vi "PCO_SetDelayExposureTime.vi"(6 "wTimeBaseExposure":u16(ring) items=["ns", "us", "ms"], 7 "wTimeBaseDelay":u16(ring) items=["ns", "us", "ms"], 8 "error in (no error)":errorcluster {"code" format="%x"}, 9 "dwExposure":u32, 10 "dwDelay":u32, 11 "ph":u64) -> (0 "error out":errorcluster {"code" format="%x"}, 2 "ErrorMessage":i32 format="%x", 3 "ph out":u64)   [LabVIEW 2019, in "SDK.lvlib" / "TimingControl.lvlib"]
doc: "<b>Description:</b>\nThis function does set the delay and exposure time and the associated time base values.\nWhen the Recording State of the camera is [run], camera timing is changed immediately (best possible), else new settings will be valid after a call of PCO_ArmCamera.\nRestrictions for the parameter values are defined through the following values in the camera description PCO_Description structure: dwMinDelayDESC, dwMaxDelayDESC, dwMinDelayStepDESC, dwMinExposDESC, dwMaxExposDESC, dwMinExposStepDESC\nDue to hardware limitations the input values cannot be set exactly for the pco.edge, pco.dimax and pco.1300 and therefore are changed to the next possible values in the camera. To retrieve the exact timing values, which are used in the pco.edge, please use function PCO_GetImageTiming.\nBecause frame rate and exposure time are also affected by the PCO_SetFrameRate command, it is strongly recommended to use either the PCO_SetFrameRate or the PCO_SetDelayExposureTime command.\n\n<b>Supported camera type:</b>\nAll cameras\n\n<b>Descriptor dependency:</b>\nNone"
uses:
  TimingControl.lvlib
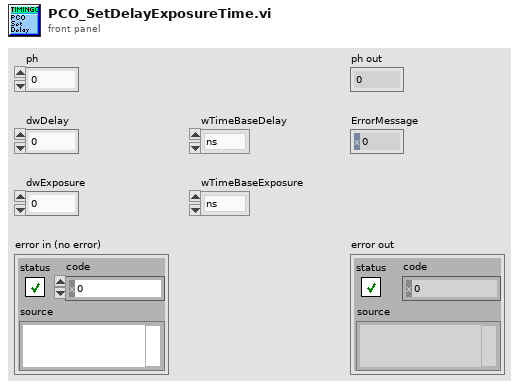
[diagram p1: front panel]
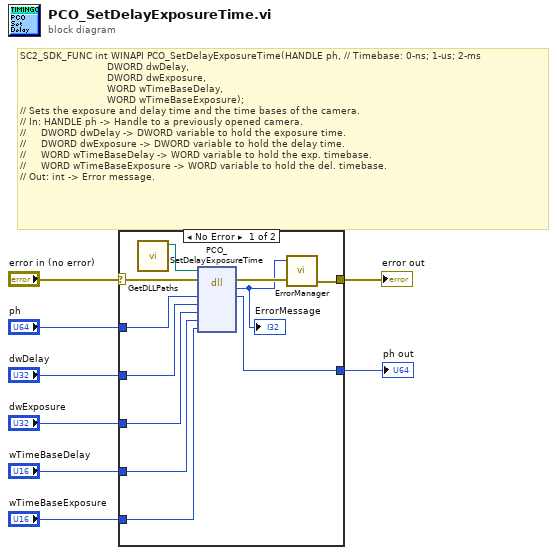
[diagram p0: block diagram]
diagram:
  # "SC2_SDK_FUNC int WINAPI PCO_SetDelayExposureTime(HANDLE ph, // Timebase: 0-ns; 1-us; 2-ms  \n                             DWORD dwDelay,\n                             DWORD dwExposure,\n                             WORD wTimeBaseDelay,\n                             WORD wTimeBaseExposure);\n// Sets the exposure and delay time and the time bases of the camera.\n// In: HANDLE ph -> Handle to a previously opened camera.\n//     DWORD dwDelay -> DWORD variable to hold the exposure time.\n//     DWORD dwExposure -> DWORD variable to hold the delay time.\n//     WORD wTimeBaseDelay -> WORD variable to hold the exp. timebase.\n//     WORD wTimeBaseExposure -> WORD variable to hold the del. timebase.\n// Out: int -> Error message."
  n1 = case shown="No Error" "error in (no error)" {
    selector: "error in (no error)" -> [w13 w20]
    tunnel: "ph" -> [w19 w21]
    tunnel: [w18 w21] -> w7
    tunnel: "dwDelay" -> [w17 _]
    tunnel: "dwExposure" -> [w16 _]
    tunnel: "wTimeBaseDelay" -> [w15 _]
    tunnel: "wTimeBaseExposure" -> [w14 _]
    tunnel: [w11 w20] -> w2
    frame No Error {
      n2 = call "GetDLLPaths.vi"() -> ("SC2_Cam_Path"=w9:path)  [unwired: 8 in, 3 out]
      n3 = dll-call lib="?" fn="PCO_SetDelayExposureTime"(path in=w9, error in=w13, "ph"=w19, "dwDelay"=w17, "dwExposure"=w16, "wTimeBaseDelay"=w15, "wTimeBaseExposure"=w14) -> (error out=w12:errorcluster, "return type"=w10:i32, "ph"=w18:u64)  [unwired: 5 in, 1 out]
      "ErrorMessage" <- w10
      n4 = call "ErrorManager.vi"("error in (no error)"=w12, "error code"=w10) -> ("error out"=w11:errorcluster)  [unwired: 2 in, 1 out]
    }
    frame Error {
    }
  }
  "ph out" <- w7
  "error out" <- w2
